vi "Parse FPGA Bitfile.vi"(8 "error in (no error)":errorcluster, 11 "Path":path) -> (0 "error out":errorcluster, 2 "DMA configuration array":T2[](array[typedef])=[{"Name"="P2PSource", "Depth"=1023, "Write? (Deprecated:Use Implementation)"=TRUE, "Physical Channel"=0, "Base Address"=65472, "Data Width"=32, "Data Type"=enum."U32", "FXP Properties"=variant(fxp<+,32,32> 0.0), "Write Window Address"=0, "Implementation"=enum."niFpgaPeerToPeerWriter", "Control Set"=0}, {"Name"="P2PSink", "Depth"=1023, "Write? (Deprecated:Use Implementation)"=FALSE, "Physical Channel"=1, "Base Address"=65408, "Data Width"=32, "Data Type"=enum."U32", "FXP Properties"=variant(fxp<+,32,32> 0.0), "Write Window Address"=57344, "Implementation"=enum."niFpgaPeerToPeerReader", "Control Set"=1}], 3 "controls":T1)   [LabVIEW 2015, in "FPGA Addon System Explorer.lvlib"]
uses:
  FPGA Addon System Explorer.lvlib
  <vilib>/rvi/FIFO/Fifo_Types/Fifo_DMA_Config.ctl
  <vilib>/rvi/DataTransferAndStorage/Container/Common/niFpgaDataTypeControl.ctl
  <vilib>/rvi/ClientSDK/Core/ModuleGeneration/CommunicationInterfaceUtility/niFpgaDmaChannelImplementation.ctl
  <vilib>/rvi/interface/common/nirviReadCallControlInfo.ctl
  <vilib>/rvi/ClientSDK/Host Interface/DMA/public/niFpgaDmaChannelVisibilityFilter.ctl
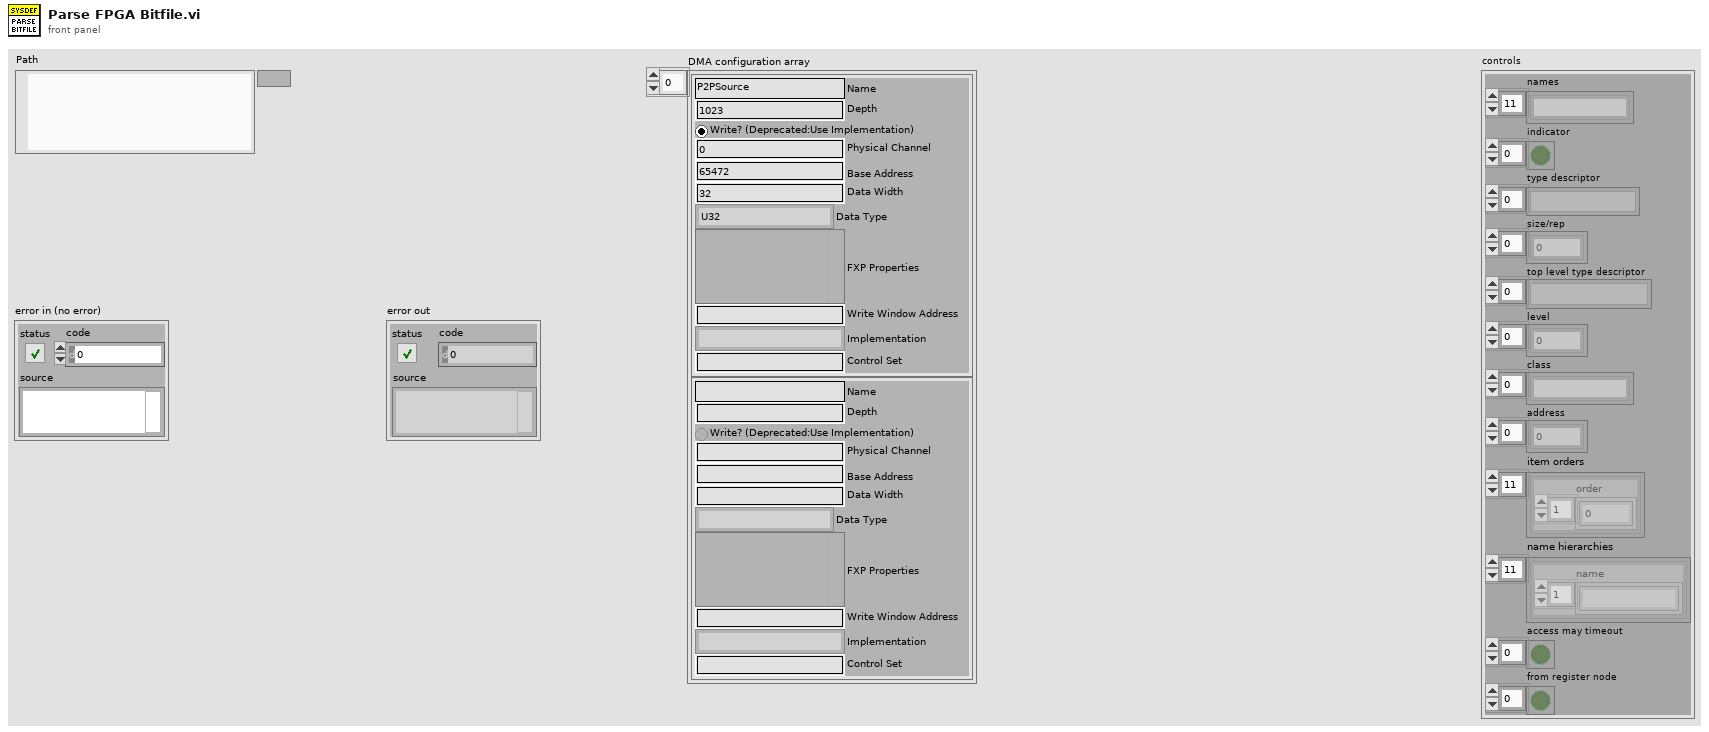
[diagram p1: front panel]
types:
  T1 = typedef "nirviReadCallControlInfo.ctl" = cluster{"names":string[], "indicator":bool[], "type descriptor":variant[], "size/rep":u32[], "top level type descriptor":variant[], "level":i32[], "class":string[], "address":i32[], "item orders":cluster{"order":u32[]}[], "name hierarchies":cluster{"name":string[]}[], "access may timeout":bool[], "from register node":bool[]}
  T2 = typedef "Fifo_DMA_Config.ctl" = cluster{"Name":string, "Depth":u32, "Write? (Deprecated:Use Implementation)":bool, "Physical Channel":u32, "Base Address":u32, "Data Width":u32, "Data Type":T3, "FXP Properties":variant, "Write Window Address":u32, "Implementation":T4, "Control Set":u32}
  T3 = typedef "niFpgaDataTypeControl.ctl" = enum32{"Boolean", "I8", "I16", "I32", "I64", "U8", "U16", "U32", "U64", "FXP", "CustomControl", "SGL"}
  T4 = typedef "niFpgaDmaChannelImplementation.ctl" = enum16{"niFpgaTargetToHost", "niFpgaHostToTarget", "niFpgaPeerToPeerWriter", "niFpgaPeerToPeerReader", "niCoreTargetToHost", "niCoreHostToTarget"}
  T5 = typedef "niFpgaDmaChannelVisibilityFilter.ctl" = enum16{"All", "UserVisible"}
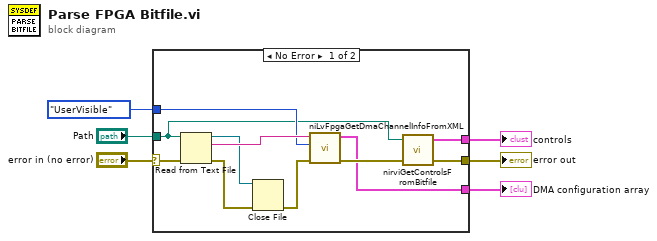
[diagram p0: block diagram]
diagram:
  n1 = case shown="No Error" "error in (no error)" {
    selector: "error in (no error)" -> [w12 w18]
    tunnel: [w9 w18] -> w5
    tunnel: "Path" -> [w10 _]
    tunnel: niFpgaDmaChannelVisibilityFilter."UserVisible" ("DMA Channel Filter") -> [w11 _]
    tunnel: [w8 _] -> w1
    tunnel: [w7 _] -> w2
    frame No Error {
      n2 = Read from Text File(file (use dialog)=w10, error in=w12) -> (refnum out=w15:refnum<file>, text=w17:string, error out=w14:errorcluster)  [unwired: 3 out]
      n3 = Close File(refnum=w15, error in=w14) -> (error out=w13:errorcluster)  [unwired: 1 out]
      n4 = call <resource>:"niLvFpgaGetDmaChannelInfoFromXML.vi"("error in (no error)"=w13, "DMA Channel Filter"=w11, "XML String in"=w17) -> ("error out"=w16:errorcluster, "DMA configuration array"=w7:T2[])  [unwired: 7 out]
      n5 = call <vilib>:"nirviGetControlsFromBitfile.vi"("error in (no error)"=w16, "bitfile path"=w10) -> ("error out"=w9:errorcluster, "controls"=w8:T1)  [unwired: 2 in]
    }
    frame Error {
    }
  }
  "error out" <- w5
  "DMA configuration array" <- w2
  "controls" <- w1
